vi "S2C_FORNAX_Poly_FeatureSettingsCommand.vi"(8 "Error In":errorcluster, 10 "FeatureSettingsCommand":T3={"Partition"="Default", "Message"="FeatureSettingsCommand", "M_FeatureCommand"=0, "M_FeatureSetting"=0, "M_IntValue"=0, "M_IsEnabled"=FALSE, "M_IsEntitled"=FALSE, "M_LicenseKey"="", "M_LicenseTerms"="", "M_Options"="", "M_StringValue"=""} {"M_FeatureSetting" items=["FEATURE_SETTINGS_INVALID", "FEATURE_SETTINGS_SOFT_COAG", "FEATURE_SETTINGS_SHARED_COAG", "FEATURE_SETTINGS_AUTOBIPOLAR", "FEATURE_SETTINGS_AMMETER", "FEATURE_SETTINGS_FX_BIPOLAR_MODES", "FEATURE_SETTINGS_CARDIOBLATE_SUPPORT", "FEATURE_SETTINGS_EINSTEIN", "FEATURE_SETTINGS_VLAB_ON_CUT_MONO1", "FEATURE_SETTINGS_VLAB_ON_CUT_MONO2", "FEATURE_SETTINGS_ENDO", "FEATURE_SETTINGS_ANIMAL_HEALTH", "FEATURE_SETTINGS_MODEL_TYPE_ES_ONLY", "FEATURE_SETTINGS_MODEL_TYPE_LS_ONLY", "FEATURE_SETTINGS_GENERAL_DATA_PROTECTION_REGULATION", "NUM_FEATURE_SETTINGS"]; "M_FeatureCommand" items=["FEATURE_SETTINGS_COMMAND_NONE", "FEATURE_SETTINGS_COMMAND_WRITE", "FEATURE_SETTINGS_COMMAND_READ", "FEATURE_SETTINGS_COMMAND_ENTITLE", "FEATURE_SETTINGS_COMMAND_REVOKE", "FEATURE_SETTINGS_COMMAND_ENABLE", "FEATURE_SETTINGS_COMMAND_DISABLE", "FEATURE_SETTINGS_COMMAND_RESTORE_TO_DEFAULT"]}, 11 "Settings":T4={"Driver"="Fornax", "Command"="FeatureSettingsCommand", "Return"="ErrorStatus", "Parameters"="", "Timeout"=10.0}) -> (0 "Error Out":errorcluster, 3 "Response":string)   [LabVIEW 2015]
uses:
  Typedefs/FeatureSettingsCommand.ctl
  Typedefs/FeatureSettings.ctl
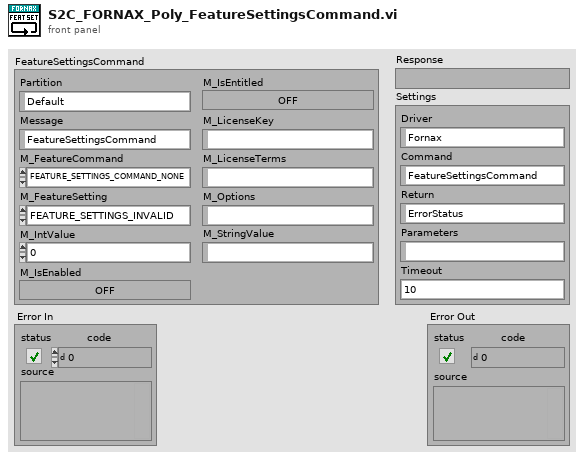
[diagram p1: front panel]
types:
  T1 = typedef "FeatureSettingsCommand.ctl" = i16
  T2 = typedef "FeatureSettings.ctl" = i16
  T3 = cluster{"Partition":string, "Message":string, "M_FeatureCommand":T1, "M_FeatureSetting":T2, "M_IntValue":i32, "M_IsEnabled":bool, "M_IsEntitled":bool, "M_LicenseKey":string, "M_LicenseTerms":string, "M_Options":string, "M_StringValue":string}
  T4 = cluster{"Driver":string, "Command":string, "Return":string, "Parameters":string, "Timeout":dbl}
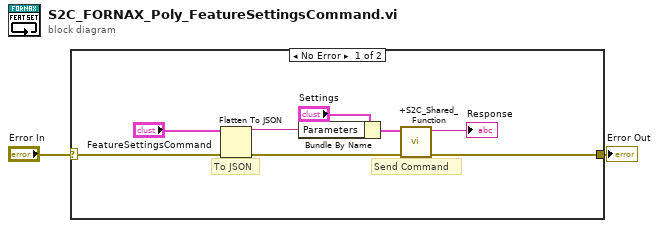
[diagram p0: block diagram]
diagram:
  n1 = case shown="No Error" "Error In" {
    selector: "Error In" -> [w6 w11]
    tunnel: [w5 w11] -> w1
    frame No Error {
      # "To JSON"
      # "Send Command"
      n2 = Flatten To JSON(anything="FeatureSettingsCommand", error in (no error)=w6) -> (JSON string=w7:string, 11:w9:errorcluster)  [unwired: 1 in]
      n3 = Bundle By Name(cluster="Settings", "Parameters"=w7) -> (w10:T4)
      n4 = call "+S2C_Shared_Function.vi"("Error In"=w9, "Settings"=w10) -> ("Error Out"=w5:errorcluster, "Response"=→"Response":string)  [unwired: 8 in]
    }
    frame Error {
    }
  }
  "Error Out" <- w1
